vi "CCD_ReadResult.vi"(8 "错误输入（无错误）":errorcluster, 10 "Input Line":string="T1", 11 "TCP网络连接输入":refnum<k5>) -> (0 "错误输出":errorcluster, 1 "数字":dbl[](array[numeric]), 2 "Array out":string[](array[string]), 3 "字符串":string, 4 "连接ID输出":refnum<k5>, 5 "CCD- TOP补正":string)   [LabVIEW 2015]
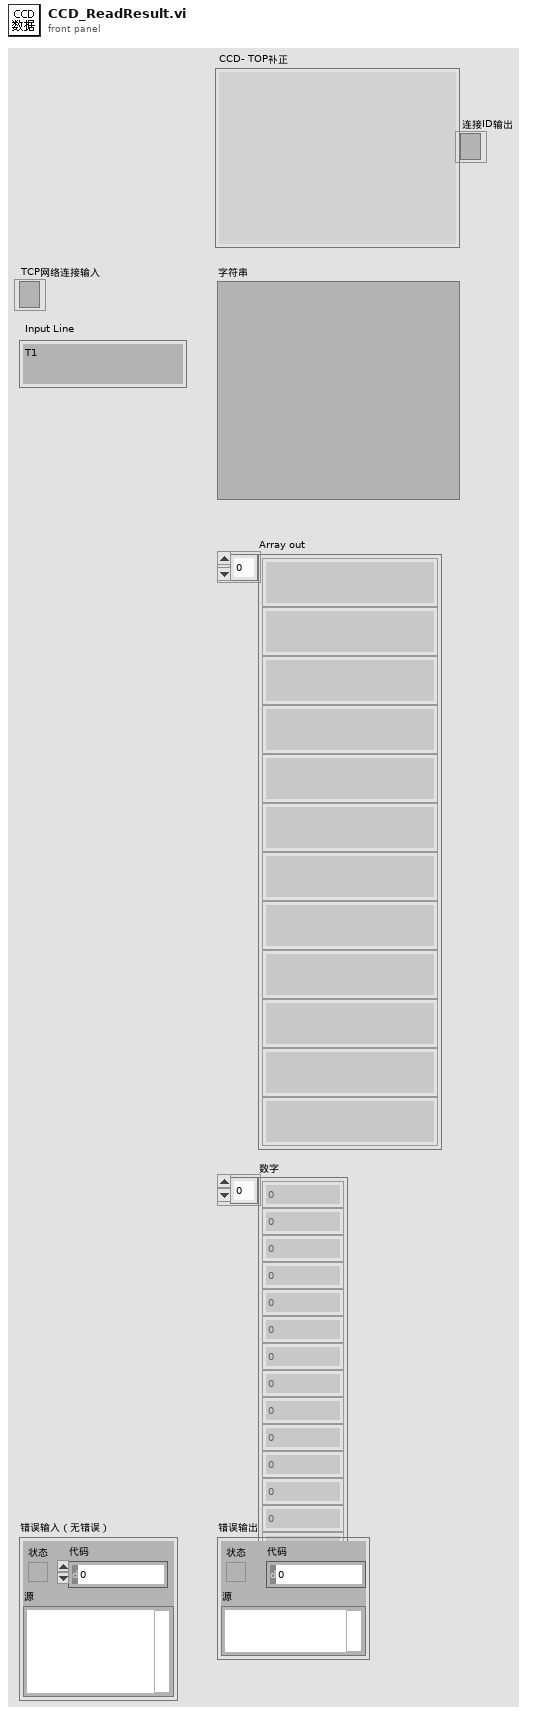
[diagram p1: front panel]
types:
  T1 = enum16{"Standard", "Buffered", "CRLF", "Immediate"}
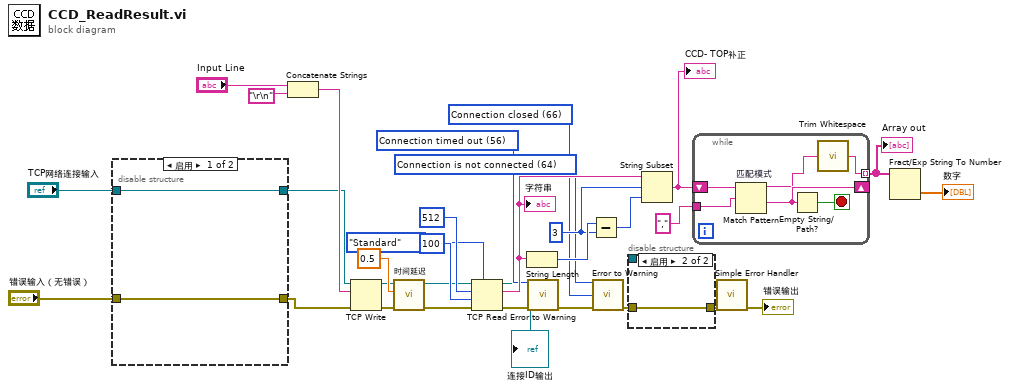
[diagram p0: block diagram]
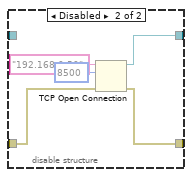
[diagram p2: hidden frame]
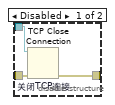
[diagram p3: hidden frame]
diagram:
  w24 = 3 ("偏移量(0)")
  w14 = 56 items=["No Error", "Argument Error", "Memory Full", "Out of Zone", "End of File", "File Already Open", "Generic File IO Error", "File Not Found", "File Permission Error", "Disk Full", "Duplicate Path", "Too Many Files Open", "Not Enabled", "Resource File Not Found", "Cannot Add Resource", "Resource Not Found", "Image Not Found", "Image Memory Error", "Pen Does Not Exist", "Config Bad Type", "Config Token Not Found", "Config Parse Error", "Config Memory Error", "Bad External Code Format", "Bad External Code Offset", "External Code Not Present", "Null Window", "Destroy Window Mixup", "Null Menu", "Print Aborted", "Bad Print Record", "Print Driver Error", "Windows Error During Print", "Memory Error During Print", "Print Dialog Error", "Generic Print Error", "Invalid Device Refnum", "Device Not Found", "Device Parameter Error", "Device Unit Error", "Can't Open Device", "Device Call Aborted", "Generic Error", "Cancelled By User", "Object ID Too Low", "Object ID Too High", "Object Not In Heap", "Unknown Heap", "Bad DefProc ID", "DefProc Not In Table", "Message Out Of Range", "Null Method", "Unknown Message", "Manager Call Not Supported", "Bad address", "Connection In progress", "Connection timed out", "Connection is already in progress", "Network attribute not supported", "Network error", "Address in use", "System out of memory", "Connection aborted", "Connection refused", "Connection is not connected", "Connection is already connected", "Connection closed", "Initialize error (interapplication manager)", "Bad occurrence", "Wait on unbound occurrence handler", "Occurrence queue overflow", "Bad path", "Semaphore not signaled", "Unrecognized type (interapplication manager)"] ("1st Error to Convert")
  w12 = 66 items=["No Error", "Argument Error", "Memory Full", "Out of Zone", "End of File", "File Already Open", "Generic File IO Error", "File Not Found", "File Permission Error", "Disk Full", "Duplicate Path", "Too Many Files Open", "Not Enabled", "Resource File Not Found", "Cannot Add Resource", "Resource Not Found", "Image Not Found", "Image Memory Error", "Pen Does Not Exist", "Config Bad Type", "Config Token Not Found", "Config Parse Error", "Config Memory Error", "Bad External Code Format", "Bad External Code Offset", "External Code Not Present", "Null Window", "Destroy Window Mixup", "Null Menu", "Print Aborted", "Bad Print Record", "Print Driver Error", "Windows Error During Print", "Memory Error During Print", "Print Dialog Error", "Generic Print Error", "Invalid Device Refnum", "Device Not Found", "Device Parameter Error", "Device Unit Error", "Can't Open Device", "Device Call Aborted", "Generic Error", "Cancelled By User", "Object ID Too Low", "Object ID Too High", "Object Not In Heap", "Unknown Heap", "Bad DefProc ID", "DefProc Not In Table", "Message Out Of Range", "Null Method", "Unknown Message", "Manager Call Not Supported", "Bad address", "Connection In progress", "Connection timed out", "Connection is already in progress", "Network attribute not supported", "Network error", "Address in use", "System out of memory", "Connection aborted", "Connection refused", "Connection is not connected", "Connection is already connected", "Connection closed", "Initialize error (interapplication manager)", "Bad occurrence", "Wait on unbound occurrence handler", "Occurrence queue overflow", "Bad path", "Semaphore not signaled", "Unrecognized type (interapplication manager)"] ("3rd Error to Convert")
  w11 = 64 items=["No Error", "Argument Error", "Memory Full", "Out of Zone", "End of File", "File Already Open", "Generic File IO Error", "File Not Found", "File Permission Error", "Disk Full", "Duplicate Path", "Too Many Files Open", "Not Enabled", "Resource File Not Found", "Cannot Add Resource", "Resource Not Found", "Image Not Found", "Image Memory Error", "Pen Does Not Exist", "Config Bad Type", "Config Token Not Found", "Config Parse Error", "Config Memory Error", "Bad External Code Format", "Bad External Code Offset", "External Code Not Present", "Null Window", "Destroy Window Mixup", "Null Menu", "Print Aborted", "Bad Print Record", "Print Driver Error", "Windows Error During Print", "Memory Error During Print", "Print Dialog Error", "Generic Print Error", "Invalid Device Refnum", "Device Not Found", "Device Parameter Error", "Device Unit Error", "Can't Open Device", "Device Call Aborted", "Generic Error", "Cancelled By User", "Object ID Too Low", "Object ID Too High", "Object Not In Heap", "Unknown Heap", "Bad DefProc ID", "DefProc Not In Table", "Message Out Of Range", "Null Method", "Unknown Message", "Manager Call Not Supported", "Bad address", "Connection In progress", "Connection timed out", "Connection is already in progress", "Network attribute not supported", "Network error", "Address in use", "System out of memory", "Connection aborted", "Connection refused", "Connection is not connected", "Connection is already connected", "Connection closed", "Initialize error (interapplication manager)", "Bad occurrence", "Wait on unbound occurrence handler", "Occurrence queue overflow", "Bad path", "Semaphore not signaled", "Unrecognized type (interapplication manager)"] ("1st Error to Convert")
  n1 = disable-structure shown="启用" {
    disable-tunnel: [w33 w36] -> w3
    disable-tunnel: "TCP网络连接输入" -> [w33 _]
    disable-tunnel: "错误输入（无错误）" -> [w32 w34]
    disable-tunnel: [w32 w35] -> w1
    frame Enabled {
    }
    frame Disabled {
      n2 = TCP Open Connection(address="192.168.0.50" ("地址"), remote port or service name=u16 8500 ("远程端口或服务名称"), error in (no error)=w34) -> (connection ID=w36:refnum<k5>, error out=w35:errorcluster)  [unwired: 2 in]
    }
  }
  n3 = Concatenate Strings("Input Line", "\r\n") -> (w23:string)
  n4 = TCP Write(connection ID=w3, data in=w23, error in (no error)=w1) -> (connection ID out=w7:refnum<k5>, error out=w19:errorcluster)  [unwired: 1 in, 1 out]
  n5 = call "时间延迟"("error in (no error)"=w19, "Delay Time (s)"=0.5) -> ("error out"=w20:errorcluster)  [unwired: 9 in]
  n6 = TCP Read(connection ID=w7, bytes to read=512, error in (no error)=w20, 7:T1."Standard" ("模式（标准）"), 9:100) -> (connection ID out=→"连接ID输出":refnum<k5>, data out=w30:string, error out=w13:errorcluster)
  "字符串" <- w30
  n7 = String Length(string=w30) -> (length=w31:i32)
  n8 = call <vilib>:"Error to Warning.vi"("1st Error to Convert"=w14, "error in"=w13) -> ("warning out"=w15:errorcluster)  [unwired: 13 in]
  n9 = Subtract(x=w31, y=w24) -> (x-y=w25:i32)
  n10 = call <vilib>:"Error to Warning.vi"("1st Error to Convert"=w11, "3rd Error to Convert"=w12, "error in"=w15) -> ("warning out"=w8:errorcluster)  [unwired: 12 in]
  n11 = disable-structure shown="启用" {
    disable-tunnel: [w41 w42] -> w9
    disable-tunnel: w8 -> [w40 w42]
    disable-tunnel: _ -> [w39 _]
    frame Disabled {
      n12 = TCP Close Connection "关闭TCP连接"(connection ID=w39, error in (no error)=w40) -> (error out=w41:errorcluster)  [unwired: 1 in, 1 out]
    }
    frame Enabled {
    }
  }
  n13 = String Subset(string=w30, offset (0)=w24, length (rest)=w25) -> (substring=w29:string)
  "CCD- TOP补正" <- w29
  n14 = while {
    tunnel: "," ("regular expression") -> [w47]
    shift-right: [w46] -> _
    shift-left: w29 -> [w48]
    tunnel: [w43] -> w27 mode=indexing
    stop <- w45 stop-if-true
    n15 = Match Pattern "匹配模式"(string=w48, regular expression=w47) -> (before substring=w44:string, after substring=w46:string)  [unwired: 1 in, 2 out]
    n16 = Empty String/Path?(string/path=w46) -> (empty?=w45:bool)
    n17 = call <vilib>:"Trim Whitespace.vi"("string"=w44) -> ("trimmed string"=w43:string)  [unwired: 1 in]
  }
  "Array out" <- w27
  n18 = call <vilib>:"Simple Error Handler.vi"("error in (no error)"=w9) -> ("error out"=→"错误输出":errorcluster)  [unwired: 4 in, 4 out]
  n19 = Fract/Exp String To Number(string=w27) -> (number=→"数字":dbl[])  [unwired: 3 in, 1 out]
